vi "Format Table Rows into Fixed Table.vi"(5 "Table Pixel Width (1800)":i16=1800, 7 "Column Pixel Widths":i16[](array[numeric]), 9 "Table Headers":string[](array[string]), 11 "Table Rows":string[](array[string])) -> (3 "Table Text":string)   [LabVIEW 2023, in "Confluence Formatting.lvlib"]
uses:
  Confluence Formatting.lvlib
  Types/Format Combo Box.ctl
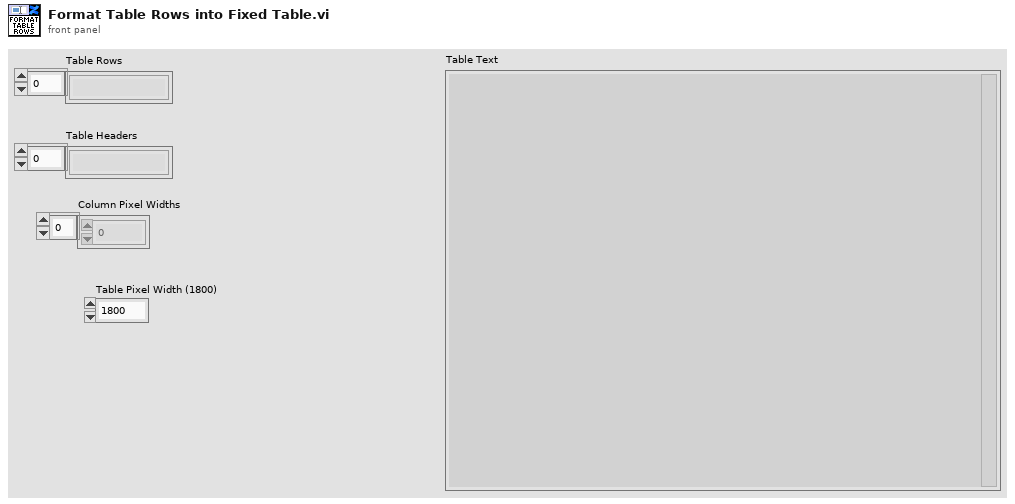
[diagram p1: front panel]
types:
  T1 = typedef "Confluence Formatting.lvlib/Format Combo Box.ctl" = string
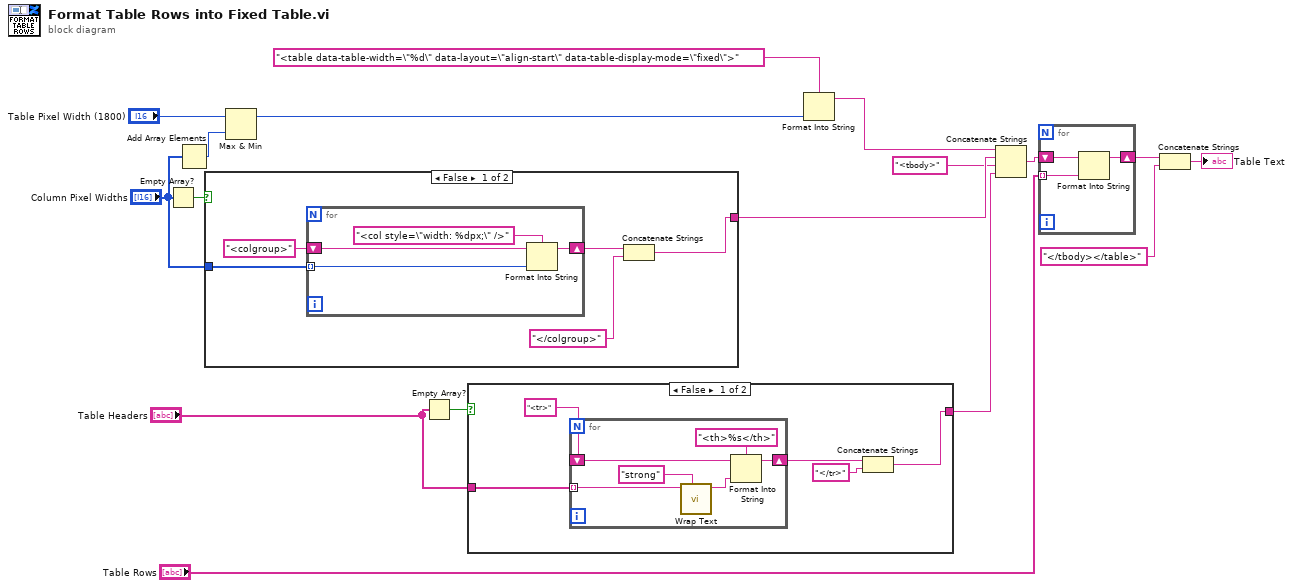
[diagram p0: block diagram]
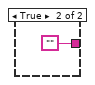
[diagram p2: hidden frame]
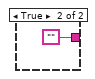
[diagram p3: hidden frame]
diagram:
  n1 = Empty Array?(array="Column Pixel Widths") -> (empty?=w9:bool)
  n2 = Add Array Elements(numeric array="Column Pixel Widths") -> (sum=w3:i16)
  n3 = case shown="False" w9 {
    tunnel: "Column Pixel Widths" -> [w21 _]
    tunnel: [w18 ""] -> w8
    frame False {
      n4 = for {
        tunnel: w21 -> [w23] mode=indexing
        shift-right: [w24] -> w19
        shift-left: "<colgroup>" -> [w26]
        n5 = Format Into String(format string="<col style=\"width: %dpx;\" />", initial string=w26, w23) -> (resulting string=w24:string)  [unwired: 1 in, 1 out]
      }
      n6 = Concatenate Strings(w19, "</colgroup>" ("string")) -> (w18:string)
    }
    frame True {
    }
  }
  n7 = Max & Min(x="Table Pixel Width (1800)", y=w3) -> (max(x,y)=w1:i16)  [unwired: 1 out]
  n8 = Empty Array?(array="Table Headers") -> (empty?=w12:bool)
  n9 = case shown="False" w12 {
    tunnel: "Table Headers" -> [w31 _]
    tunnel: [w28 ""] -> w10
    frame False {
      n10 = for {
        tunnel: w31 -> [w38] mode=indexing
        shift-right: [w33] -> w29
        shift-left: "<tr>" -> [w35]
        n11 = call "Wrap Text.vi"("Formatting"=T1 "strong", "String"=w38) -> ("Wrapped String"=w36:string)  [unwired: 8 in, 1 out]
        n12 = Format Into String(format string="<th>%s</th>", initial string=w35, w36) -> (resulting string=w33:string)  [unwired: 1 in, 1 out]
      }
      n13 = Concatenate Strings(w29, "</tr>" ("string")) -> (w28:string)
    }
    frame True {
    }
  }
  n14 = Format Into String(format string="<table data-table-width=\"%d\" data-layout=\"align-start\" data-table-display-mode=\"fixed\">", w1) -> (resulting string=w5:string)  [unwired: 2 in, 1 out]
  n15 = Concatenate Strings(w5, w8, "<tbody>" ("string"), w10) -> (w11:string)
  n16 = for {
    tunnel: "Table Rows" -> [w41] mode=indexing
    shift-right: [w40] -> w16
    shift-left: w11 -> [w42]
    n17 = Format Into String(initial string=w42, w41) -> (resulting string=w40:string)  [unwired: 2 in, 1 out]
  }
  n18 = Concatenate Strings(w16, "</tbody></table>" ("string")) -> (→"Table Text":string)
